vi "templates delete template.vi"(8 "error in (no error)":errorcluster, 10 "sxTemplateId (\"\")":string, 11 "Connection Refnum In\n(0,0: Open New)":T1) -> (0 "error out":errorcluster, 3 "Connection Refnum In\n(0,0: Open New)":T1)   [LabVIEW 2011]
uses:
  SI.LIB/ODBC/SQL Controls/Connection Refnum.ctl
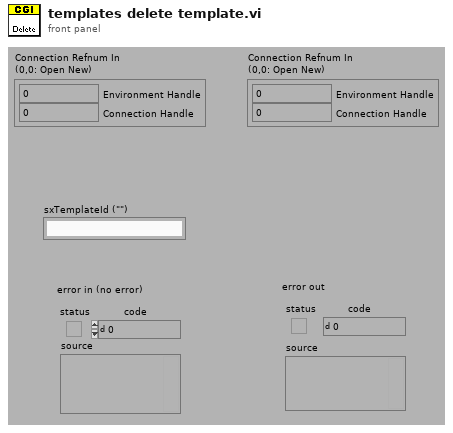
[diagram p1: front panel]
types:
  T1 = typedef "Connection Refnum.ctl" = cluster{"Environment Handle":i32, "Connection Handle":i32}
  T2 = typedef "Template Record.ctl" = cluster{"ixTemplate":i32, "sxTemplateId":string, "sDescription":string, "sCreator":string, "tCreationDate":timestamp, "sModifier":string, "tModifiedDate":timestamp, "sType":string, "sStyle":string, "sFormat":string, "dWidth":dbl, "dHeight":dbl, "sFilename":string, "sScript":string, "sLayout":string, "sEditor":string, "sStyleProcess":string}
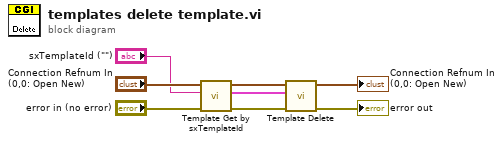
[diagram p0: block diagram]
diagram:
  n1 = call "Template Get by sxTemplateId.vi"("error in (no error)"="error in (no error)", "sxTemplateId (\"\")"="sxTemplateId (\"\")", "Connection Refnum"="Connection Refnum In\n(0,0: Open New)") -> ("error out"=w5:errorcluster, "Template Record"=w4:T2, "Connection Refnum"=w3:T1)  [unwired: 6 out]
  n2 = call "Template Delete.vi"("error in (no error)"=w5, "Template Record"=w4, "Connection Refnum"=w3) -> ("error out"=→"error out":errorcluster, "Connection Refnum"=→"Connection Refnum In\n(0,0: Open New)":T1)  [unwired: 7 out]
